vi "Main.vi"(9 "Device":string, 10 "VISA Com Port":refnum<visa-resource-name>, 11 "Module Admin":refnum<class "Delacor_lib_QMH_Cloneable Module Admin.lvclass">) -> ()   [LabVIEW 2020, in "Serial Device.lvlib"]
doc: "This template is based off of the Queued Message Handler design pattern and the Queued Message Handler project template that ships with LabVIEW.\n\nThe main difference is that the queue is private to this module and communication between modules is performed via Broadcast and Request events.\n\nRequest events are wrapped in public API methods and are handled in the Event Handling Loop (EHL) of this VI. Any module can register for Broadcast events sent by this module. The EHL generates messages based on user interface actions.\n\nThe Message Handling Loop (MHL) processes messages generated by the EHL, or by other messages. The messages are string values, so new messages can be added easily to the Message Cases case structure in the MHL. Each message cluster can also provide an optional value for Message Data, which is a variant that can be converted to whatever message-specific data is required.\n_____\nBased on Delacor QMH Project Template 5.0.0.82."
uses:
  Serial Device.lvlib
  <vilib>/Delacor/Delacor QMH/Libraries/Cloneable Module Admin_class/Delacor_lib_QMH_Cloneable Module Admin.lvclass
  C:/Program Files (x86)/National Instruments/LabVIEW 2020/vi.lib/Delacor/Delacor QMH/Libraries/Module Admin_class/Delacor_lib_QMH_Module Admin.lvclass
  Module Data--cluster.ctl
  <vilib>/Delacor/Delacor QMH/Libraries/Cloneable Module Admin_class/Delacor_lib_QMH_Cloneable Module Admin.lvclass/Delacor_lib_QMH_Cloneable Module Admin.ctl
  Stop Argument--cluster.ctl
  <vilib>/Delacor/Delacor QMH/Libraries/Message Queue_class/Delacor_lib_QMH_Message Queue.lvclass/Delacor_lib_QMH_Message Queue.ctl
  <vilib>/Delacor/Delacor QMH/Libraries/Module Admin_class/Delacor_lib_QMH_Module Admin.lvclass/Delacor_lib_QMH_Module Admin.ctl
  Write Port Argument--cluster.ctl
  Write Port (Reply Payload)--cluster.ctl
  Write Pin Argument--cluster.ctl
  Write Pin (Reply Payload)--cluster.ctl
  Read ADC Argument--cluster.ctl
  Read ADC (Reply Payload)--cluster.ctl
  Read Port Argument--cluster.ctl
  Read Port (Reply Payload)--cluster.ctl
  Read Pin Argument--cluster.ctl
  Read Pin (Reply Payload)--cluster.ctl
  Implementations/Cypress/Cypress.lvclass
  C:/Users/Asus/Dropbox/trabajos_apuntes/7 semestre/labview/Serial Device/Abstract/Serial Device/Serial Device.lvclass
  Implementations/Arduino/Arduino.lvclass
  Implementations/TI/TI.lvclass
  Implementations/Simulado/Simulado.lvclass
  Implementations/NXP/NXP.lvclass
  <vilib>/Utility/miscctls.llb/LVPointTypeDef.ctl
  <vilib>/Delacor/Delacor QMH/Libraries/Cloneable Module Admin_class/Delacor_lib_QMH_Get Module ID.vi
  <vilib>/Delacor/Delacor QMH/Libraries/Message Queue_class/Delacor_lib_QMH_Enqueue Message (Single).vi
  <vilib>/Delacor/Delacor QMH/Libraries/Module Admin_class/Delacor_lib_QMH_Get External Launch.vi
  <vilib>/Utility/error.llb/Error Cluster From Error Code.vi
  <vilib>/ErrorRing/Error Ring.xnode
  <vilib>/Delacor/Delacor QMH/Libraries/Message Queue_class/Delacor_lib_QMH_Message Queue.lvclass
  Abstract/Serial Device/Serial Device.lvclass
panel:
  out "Device Response":string
  in  "Read ADC":bool
  in  "Channel":dbl
  in  "Set Port":bool
  in  "Value":string="00"
  in  "Port":dbl
  out "Array":bool[](array[boolean])
  in  "Read Port":bool
  in  "Port 2":dbl caption="Port"
  in  "I/O Value":bool
  in  "Pin":dbl
  in  "Set PIN":bool
  in  "Port 3":dbl caption="Port"
  out "error out":errorcluster
  out "Pin Value":bool
  in  "Read PIN":bool
  in  "Pin 2":dbl caption="Pin"
  in  "Port 4":dbl caption="Port"
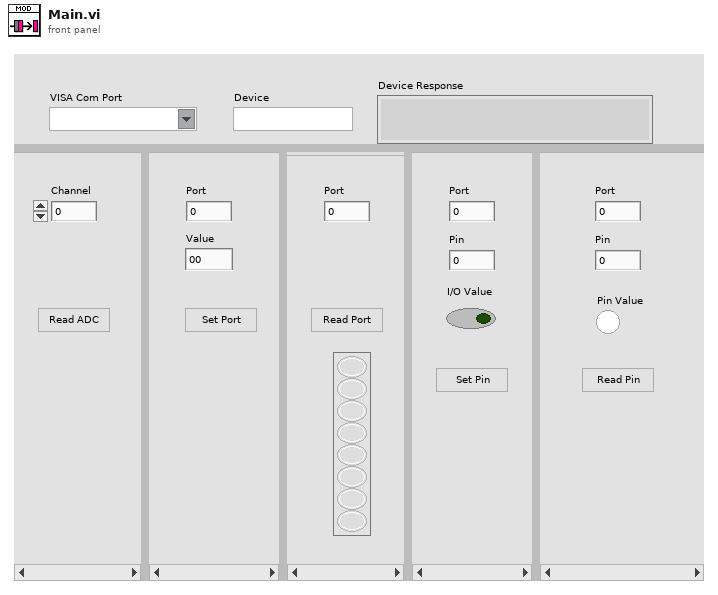
[diagram p1: front panel]
types:
  T1 = typedef "Serial Device.lvlib/Request Events--cluster.ctl" = cluster{"Stop Module":refnum<user-event>, "Show Panel":refnum<user-event>, "Hide Panel":refnum<user-event>, "Show Diagram":refnum<user-event>, "Get Module Execution Status":refnum<user-event>, "Write Port":refnum<user-event>, "Write Pin":refnum<user-event>, "Read ADC":refnum<user-event>, "Read Port":refnum<user-event>, "Read Pin":refnum<user-event>}
  T2 = typedef "Serial Device.lvlib/Module Data--cluster.ctl" = cluster{"Status":string}
  T3 = enum32{"invalid lock state", "Not Locked", "Locked (No Password)", "Password-protected"}
  T4 = typedef "Serial Device.lvlib/Stop Argument--cluster.ctl" = cluster{"Module ID":i32, "Origin":string, "Exit via Stop Module Req?":bool, "Wait for Module to stop?":bool}
  T5 = typedef "Serial Device.lvlib/Write Port Argument--cluster.ctl" = cluster{"Module ID":i32, "PORT":dbl, "VAL":string, "Wait Notifier":refnum<notifier>, "wait for reply":bool}
  T6 = typedef "Serial Device.lvlib/Write Pin Argument--cluster.ctl" = cluster{"Module ID":i32, "Port":dbl, "Value":bool, "Pin":dbl, "Wait Notifier":refnum<notifier>, "wait for reply":bool}
  T7 = typedef "Serial Device.lvlib/Read ADC Argument--cluster.ctl" = cluster{"Module ID":i32, "Channel":dbl, "Wait Notifier":refnum<notifier>, "wait for reply":bool}
  T8 = typedef "Serial Device.lvlib/Read Port Argument--cluster.ctl" = cluster{"Module ID":i32, "Port to read":dbl, "Wait Notifier":refnum<notifier>, "wait for reply":bool}
  T9 = typedef "Serial Device.lvlib/Read Pin Argument--cluster.ctl" = cluster{"Module ID":i32, "Port 4":dbl, "Pin 2":dbl, "Pin Value":bool, "Wait Notifier":refnum<notifier>, "wait for reply":bool}
  T10 = enum32{"Invalid", "Standard", "Closed", "Hidden", "Minimized", "Maximized"}
  T11 = typedef "Serial Device.lvlib/Write Port (Reply Payload)--cluster.ctl" = cluster{"Write Port_error":errorcluster, "Response":string}
  T12 = typedef "Serial Device.lvlib/Write Pin (Reply Payload)--cluster.ctl" = cluster{"Write Pin_error":errorcluster, "Response":string}
  T13 = typedef "Serial Device.lvlib/Read ADC (Reply Payload)--cluster.ctl" = cluster{"Read ADC_error":errorcluster, "Response":string}
  T14 = typedef "Serial Device.lvlib/Read Port (Reply Payload)--cluster.ctl" = cluster{"Read Port_error":errorcluster, "Response":string}
  T15 = typedef "Serial Device.lvlib/Read Pin (Reply Payload)--cluster.ctl" = cluster{"Read Pin_error":errorcluster, "Response":string}
  T16 = typedef "LVPointTypeDef.ctl" = cluster{"Horizontal":i16, "Vertical":i16}
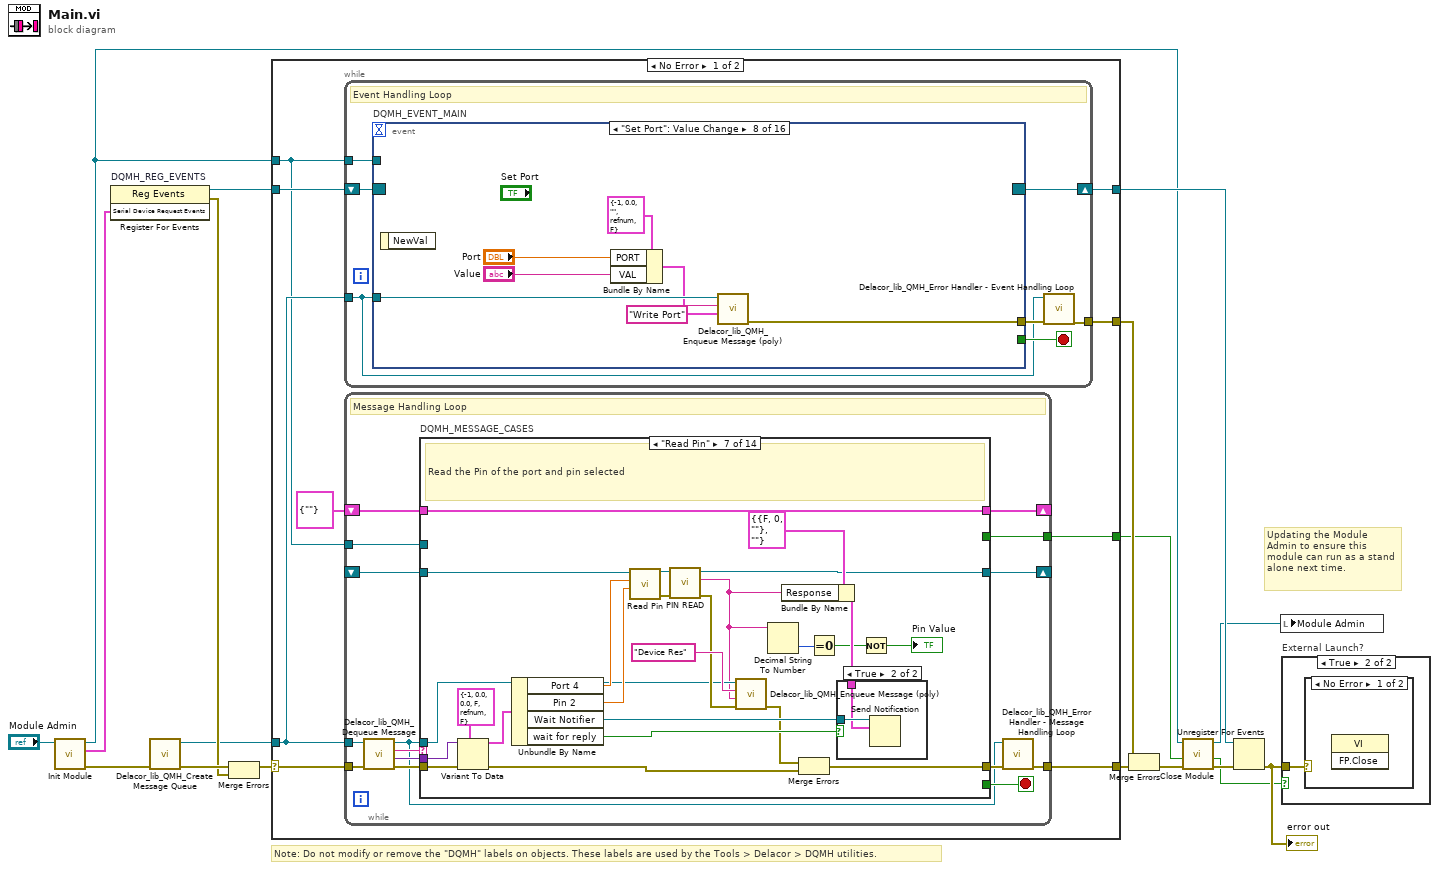
[diagram p0: block diagram]
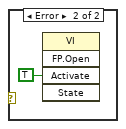
[diagram p3: hidden frame]
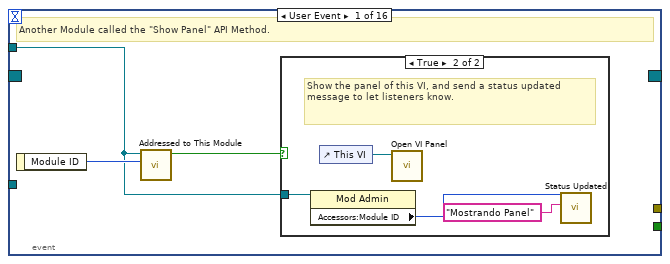
[diagram p4: hidden frame]
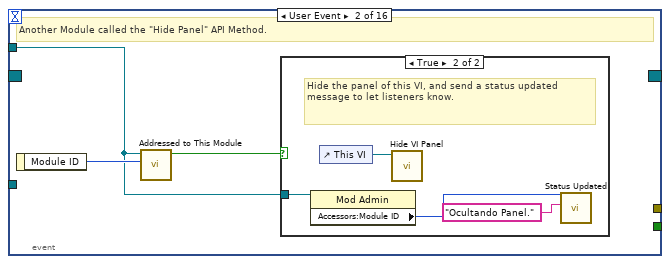
[diagram p6: hidden frame]
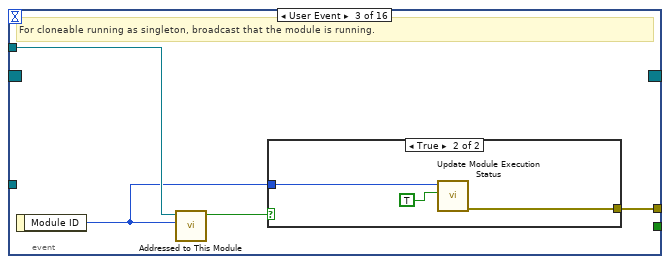
[diagram p8: hidden frame]
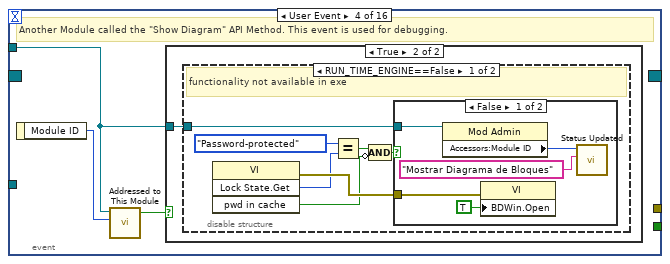
[diagram p10: hidden frame]
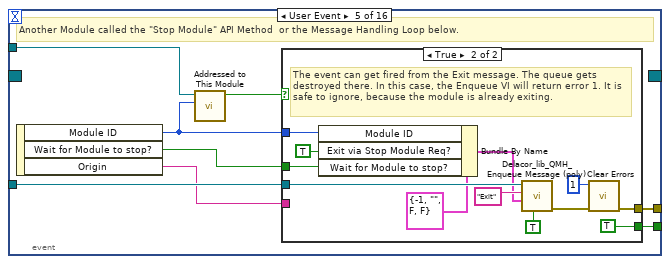
[diagram p14: hidden frame]
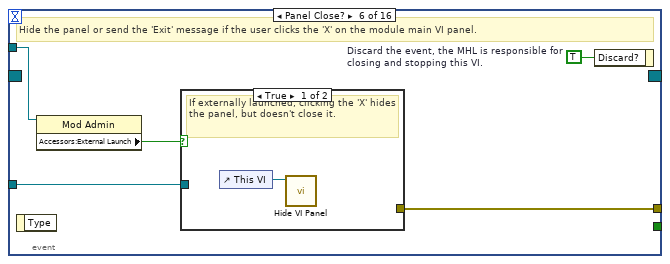
[diagram p16: hidden frame]
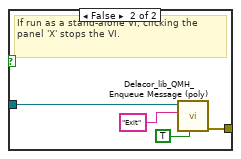
[diagram p17: hidden frame]
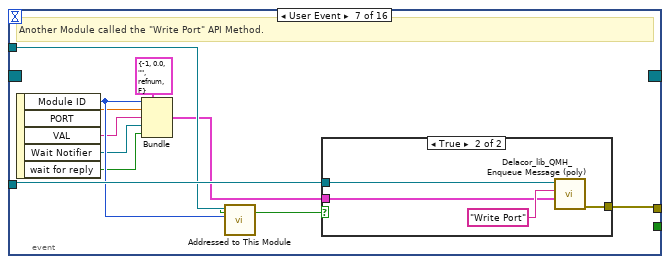
[diagram p18: hidden frame]
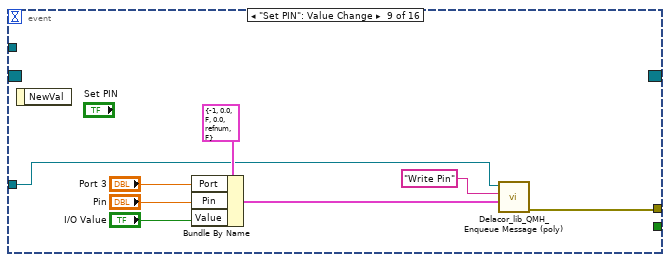
[diagram p20: hidden frame]
diagram:
  # "Note: Do not modify or remove the \"DQMH\" labels on objects. These labels are used by the Tools > Delacor > DQMH utilities."
  # "Updating the Module Admin to ensure this module can run as a stand alone next time."
  n1 = call "Init Module.vi"("Cloneable Module Admin in"="Module Admin") -> ("error out"=w15:errorcluster, "Serial Device Request Events"=w7:T1, "Cloneable Module Admin out"=w4:refnum<class "Delacor_lib_QMH_Cloneable Module Admin.lvclass">)  [unwired: 8 in]
  n2 = register-events "DQMH_REG_EVENTS"(w7) -> (reference out=w8:refnum<event-registration>, error out=w10:errorcluster)  [unwired: 2 in]
  n3 = call <vilib>:"Delacor_lib_QMH_Create Message Queue.vi"("error in (no error)"=w15) -> ("error out"=w12:errorcluster, "Message Queue"=w6:refnum<class "Delacor_lib_QMH_Message Queue.lvclass">)  [unwired: 9 in]
  n4 = Merge Errors(w12, w10) -> (w11:errorcluster)
  n5 = case shown="No Error" w11 {
    selector: w11 -> [w25 w478]
    tunnel: [w27 w477] -> w16
    tunnel: [w24 w485] -> w9
    tunnel: w8 -> [w22 w485]
    tunnel: w6 -> [w21 w476]
    tunnel: [w26 _] -> w17
    tunnel: w4 -> [w20 w481]
    tunnel: [w19 _] -> w2
    frame No Error {
      n6 = while {
        tunnel: w21 -> [w28]
        shift-right: [w31] -> w24
        shift-left: w22 -> [w32]
        tunnel: [w33] -> w26
        tunnel: w20 -> [w29]
        stop <- w30 stop-if-true
        # "Event Handling Loop"
        n7 = event "DQMH_EVENT_MAIN" shown="[7] \"Set Port\": Value Change" {
          selector: w32 -> [_ _ _ _ _ _ _ _ _ _ _ _ _ _ _ _]
          dyn-events: [_ _ _ _ _ _ _ _ _ _ _ _ _ _ _ _] -> w31
          timeout: _ -> [_ _ _ _ _ _ _ _ _ _ _ _ _ _ _ _]
          tunnel: [_ _ _ _ w75 _ _ _ _ _ _ _ _ _ _ _] -> w30
          tunnel: w28 -> [_ _ _ _ w78 w93 w112 w123 w126 w143 w157 w164 w177 w183 w190 w206]
          tunnel: [_ _ w52 _ w79 w96 w105 w122 w124 w134 w150 w163 w170 w184 w189 w197] -> w34
          tunnel: w29 -> [w35 w42 w50 w56 w77 w94 w111 _ _ w141 w155 _ w175 _ _ w204]
          event User Event {
            # "Another Module called the \"Show Panel\" API Method."
            n8 = event-data() -> ("Module ID"=w36:i32)  [unwired: 1 in]
            n9 = call "Addressed to This Module.vi"("Module ID from Argument"=w36, "Module Admin"=w35) -> ("Addressed to this instance?"=w37:bool)  [unwired: 8 in, 1 out]
            n10 = case shown="True" w37 {
              tunnel: w35 -> [_ w39]
              frame False {
              }
              frame True {
                # "Show the panel of this VI, and send a status updated message to let listeners know."
                n11 = property class="Mod Admin"(reference=w39) -> ("Accessors:Module ID"=w38:i32)  [unwired: 1 in, 2 out]
                n12 = control-ref of="This VI"() -> (w41:refnum<vi>)
                n13 = call "Open VI Panel.vi"("VI"=w41) -> ()  [unwired: 10 in, 1 out]
                n14 = call "Status Updated.vi"("Status"="Mostrando Panel" ("format string"), "Module ID"=w38) -> ()  [unwired: 9 in, 1 out]
              }
            }
          }
          event User Event {
            # "Another Module called the \"Hide Panel\" API Method."
            n15 = event-data() -> ("Module ID"=w43:i32)  [unwired: 1 in]
            n16 = call "Addressed to This Module.vi"("Module ID from Argument"=w43, "Module Admin"=w42) -> ("Addressed to this instance?"=w44:bool)  [unwired: 8 in, 1 out]
            n17 = case shown="True" w44 {
              tunnel: w42 -> [_ w46]
              frame False {
              }
              frame True {
                # "Hide the panel of this VI, and send a status updated message to let listeners know."
                n18 = property class="Mod Admin"(reference=w46) -> ("Accessors:Module ID"=w45:i32)  [unwired: 1 in, 2 out]
                n19 = control-ref of="This VI"() -> (w48:refnum<vi>)
                n20 = call "Hide VI Panel.vi"("VI"=w48) -> ()  [unwired: 10 in, 1 out]
                n21 = call "Status Updated.vi"("Status"="Ocultando Panel." ("format string"), "Module ID"=w45) -> ()  [unwired: 9 in, 1 out]
              }
            }
          }
          event User Event {
            # "For cloneable running as singleton, broadcast that the module is running."
            n22 = event-data() -> ("Module ID"=w49:i32)  [unwired: 1 in]
            n23 = call "Addressed to This Module.vi"("Module ID from Argument"=w49, "Module Admin"=w50) -> ("Addressed to this instance?"=w51:bool)  [unwired: 8 in, 1 out]
            n24 = case shown="True" w51 {
              tunnel: [_ w55] -> w52
              tunnel: w49 -> [_ w54]
              frame False {
              }
              frame True {
                n25 = call "Update Module Execution Status.vi"("Running?"=TRUE, "Module ID"=w54) -> ("error out"=w55:errorcluster)  [unwired: 9 in]
              }
            }
          }
          event User Event {
            # "Another Module called the \"Show Diagram\" API Method. This event is used for debugging."
            n26 = event-data() -> ("Module ID"=w57:i32)  [unwired: 1 in]
            n27 = call "Addressed to This Module.vi"("Module ID from Argument"=w57, "Module Admin"=w56) -> ("Addressed to this instance?"=w58:bool)  [unwired: 8 in, 1 out]
            n28 = case shown="True" w58 {
              tunnel: w56 -> [_ w59]
              frame False {
              }
              frame True {
                n29 = disable-structure shown="RUN_TIME_ENGINE==False" {
                  disable-tunnel: w59 -> [w60 _]
                  frame condition #0 (active) {
                    # "functionality not available in exe"
                    n30 = invoke class="VI" method="Lock State.Get"() -> (error out=w66:errorcluster, "Get Lock State"=w65:T3, "pwd in cache"=w62:bool)  [unwired: 4 in, 1 out]
                    n31 = Equal?(x=T3."Password-protected", y=w65) -> (x = y?=w63:bool)
                    n32 = Compound Arithmetic op=AND(w63, invert w62) -> (w61:bool)
                    n33 = case shown="False" w61 {
                      tunnel: w66 -> [w71 _]
                      tunnel: w60 -> [w68 _]
                      frame False {
                        n34 = property class="Mod Admin"(reference=w68) -> ("Accessors:Module ID"=w67:i32)  [unwired: 1 in, 2 out]
                        n35 = property class="VI"(error in=w71, "BDWin.Open"=TRUE ("Block Diagram Window:Open")) -> ()  [unwired: 1 in, 2 out]
                        n36 = call "Status Updated.vi"("Status"="Mostrar Diagrama de Bloques" ("format string"), "Module ID"=w67) -> ()  [unwired: 9 in, 1 out]
                      }
                      frame True {
                        # "Password-protected VI, and the password is not in the cache. Do not show the diagram."
                      }
                    }
                  }
                  frame condition #1 {
                  }
                }
              }
            }
          }
          event User Event {
            # "Another Module called the \"Stop Module\" API Method  or the Message Handling Loop below."
            n37 = event-data() -> ("Module ID"=w73:i32, "Wait for Module to stop?"=w74:bool, "Origin"=w72:string)  [unwired: 1 in]
            n38 = call "Addressed to This Module.vi"("Module ID from Argument"=w73, "Module Admin"=w77) -> ("Addressed to this instance?"=w76:bool)  [unwired: 8 in, 1 out]
            n39 = case shown="True" w76 {
              tunnel: [_ w90] -> w79
              tunnel: w78 -> [_ w86]
              tunnel: [_ TRUE] -> w75
              tunnel: w74 -> [_ w81]
              tunnel: w73 -> [_ w83]
              tunnel: w72 -> [_ _]
              frame False {
              }
              frame True {
                # "The event can get fired from the Exit message. The queue gets destroyed there. In this case, the Enqueue VI will return error 1. It is safe to ignore, because the module is already exiting."
                n40 = Bundle By Name(cluster=T4 {"Module ID"=-1, "Origin"="", "Exit via Stop Module Req?"=FALSE, "Wait for Module to stop?"=FALSE} ("Stop Argument"), "Module ID"=w83, "Exit via Stop Module Req?"=TRUE, "Wait for Module to stop?"=w81) -> (w80:T4)
                n41 = call-poly <vilib>:"Delacor_lib_QMH_Enqueue Message (poly).vi"("Priority Message? (F)"=TRUE, "Message Data"=w80, "Message"="Exit", "Message Queue in"=w86) -> ("error out"=w91:errorcluster)  [unwired: 6 in, 1 out]
                n42 = call <vilib>:"Clear Errors.vi"("error in (no error)"=w91, "specific error code to clear (0: all)"=1) -> ("error out"=w90:errorcluster)  [unwired: 4 in, 1 out]
              }
            }
          }
          event Panel Close? {
            w95 = TRUE  # Discard the event, the MHL is responsible for closing and stopping this VI.
            # "Hide the panel or send the 'Exit' message if the user clicks the 'X' on the module main VI panel."
            n43 = event-data() -> ()  [unwired: 1 in, 1 out]
            n44 = property class="Mod Admin"(reference=w94) -> ("Accessors:External Launch"=w92:bool)  [unwired: 1 in, 2 out]
            n45 = case shown="True" w92 {
              tunnel: w93 -> [_ w100]
              tunnel: [_ w101] -> w96
              frame True {
                # "If externally launched, clicking the 'X' hides the panel, but doesn't close it."
                n46 = control-ref of="This VI"() -> (w97:refnum<vi>)
                n47 = call "Hide VI Panel.vi"("VI"=w97) -> ()  [unwired: 10 in, 1 out]
              }
              frame False {
                # "If run as a stand-alone VI, clicking the panel 'X' stops the VI."
                n48 = call-poly <vilib>:"Delacor_lib_QMH_Enqueue Message (poly).vi"("Priority Message? (F)"=TRUE, "Message"="Exit", "Message Queue in"=w100) -> ("error out"=w101:errorcluster)  [unwired: 7 in, 1 out]
              }
            }
            n49 = event-data("Discard?"=w95) -> ()  [unwired: 1 in, 1 out]
          }
          event User Event {
            # "Another Module called the \"Write Port\" API Method."
            n50 = event-data() -> ("Module ID"=w108:i32, "PORT"=w107:dbl, "VAL"=w106:string, "Wait Notifier"=w104:refnum<notifier>, "wait for reply"=w103:bool)  [unwired: 1 in]
            n51 = Bundle(cluster=T5 {"Module ID"=-1, "PORT"=0.0, "VAL"="", "Wait Notifier"=refnum, "wait for reply"=FALSE} ("Write Port Argument"), "Module ID"=w108, "PORT"=w107, "VAL"=w106, "Wait Notifier"=w104, "wait for reply"=w103) -> (w109:T5)
            n52 = call "Addressed to This Module.vi"("Module ID from Argument"=w108, "Module Admin"=w111) -> ("Addressed to this instance?"=w102:bool)  [unwired: 8 in, 1 out]
            n53 = case shown="True" w102 {
              tunnel: w112 -> [_ w116]
              tunnel: w109 -> [_ w114]
              tunnel: [_ w113] -> w105
              frame False {
              }
              frame True {
                n54 = call-poly <vilib>:"Delacor_lib_QMH_Enqueue Message (poly).vi"("Message Data"=w114, "Message"="Write Port", "Message Queue in"=w116) -> ("error out"=w113:errorcluster)  [unwired: 7 in, 1 out]
              }
            }
          }
          event "Set Port": Value Change {
            n55 = event-data() -> ()  [unwired: 1 in, 1 out]
            n56 = Bundle By Name(cluster=T5 {"Module ID"=-1, "PORT"=0.0, "VAL"="", "Wait Notifier"=refnum, "wait for reply"=FALSE} ("Write Port Argument"), "PORT"="Port", "VAL"="Value") -> (w120:T5)
            n57 = call-poly <vilib>:"Delacor_lib_QMH_Enqueue Message (poly).vi"("Message Data"=w120, "Message"="Write Port", "Message Queue in"=w123) -> ("error out"=w122:errorcluster)  [unwired: 7 in, 1 out]
          }
          event "Set PIN": Value Change {
            n58 = event-data() -> ()  [unwired: 1 in, 1 out]
            n59 = Bundle By Name(cluster=T6 {"Module ID"=-1, "Port"=0.0, "Value"=FALSE, "Pin"=0.0, "Wait Notifier"=refnum, "wait for reply"=FALSE} ("Write Pin Argument"), "Port"="Port 3", "Pin"="Pin", "Value"="I/O Value") -> (w125:T6)
            n60 = call-poly <vilib>:"Delacor_lib_QMH_Enqueue Message (poly).vi"("Message Data"=w125, "Message"="Write Pin", "Message Queue in"=w126) -> ("error out"=w124:errorcluster)  [unwired: 7 in, 1 out]
          }
          event User Event {
            # "Another Module called the \"Write Pin\" API Method."
            n61 = event-data() -> ("Module ID"=w138:i32, "Port"=w137:dbl, "Value"=w136:bool, "Pin"=w135:dbl, "Wait Notifier"=w133:refnum<notifier>, "wait for reply"=w132:bool)  [unwired: 1 in]
            n62 = Bundle(cluster=T6 {"Module ID"=-1, "Port"=0.0, "Value"=FALSE, "Pin"=0.0, "Wait Notifier"=refnum, "wait for reply"=FALSE} ("Write Pin Argument"), "Module ID"=w138, "Port"=w137, "Value"=w136, "Pin"=w135, "Wait Notifier"=w133, "wait for reply"=w132) -> (w139:T6)
            n63 = call "Addressed to This Module.vi"("Module ID from Argument"=w138, "Module Admin"=w141) -> ("Addressed to this instance?"=w142:bool)  [unwired: 8 in, 1 out]
            n64 = case shown="True" w142 {
              tunnel: w143 -> [_ w147]
              tunnel: w139 -> [_ w145]
              tunnel: [_ w144] -> w134
              frame False {
              }
              frame True {
                n65 = call-poly <vilib>:"Delacor_lib_QMH_Enqueue Message (poly).vi"("Message Data"=w145, "Message"="Write Pin", "Message Queue in"=w147) -> ("error out"=w144:errorcluster)  [unwired: 7 in, 1 out]
              }
            }
          }
          event User Event {
            # "Another Module called the \"Read ADC\" API Method."
            n66 = event-data() -> ("Module ID"=w152:i32, "Channel"=w151:dbl, "Wait Notifier"=w149:refnum<notifier>, "wait for reply"=w148:bool)  [unwired: 1 in]
            n67 = Bundle(cluster=T7 {"Module ID"=-1, "Channel"=0.0, "Wait Notifier"=refnum, "wait for reply"=FALSE} ("Read ADC Argument"), "Module ID"=w152, "Channel"=w151, "Wait Notifier"=w149, "wait for reply"=w148) -> (w153:T7)
            n68 = call "Addressed to This Module.vi"("Module ID from Argument"=w152, "Module Admin"=w155) -> ("Addressed to this instance?"=w156:bool)  [unwired: 8 in, 1 out]
            n69 = case shown="True" w156 {
              tunnel: w157 -> [_ w161]
              tunnel: w153 -> [_ w159]
              tunnel: [_ w158] -> w150
              frame False {
              }
              frame True {
                n70 = call-poly <vilib>:"Delacor_lib_QMH_Enqueue Message (poly).vi"("Message Data"=w159, "Message"="Read ADC", "Message Queue in"=w161) -> ("error out"=w158:errorcluster)  [unwired: 7 in, 1 out]
              }
            }
          }
          event "Read ADC": Value Change {
            n71 = event-data() -> ()  [unwired: 1 in, 1 out]
            n72 = Bundle By Name(cluster=T7 {"Module ID"=-1, "Channel"=0.0, "Wait Notifier"=refnum, "wait for reply"=FALSE} ("Read ADC Argument"), "Channel"="Channel") -> (w162:T7)
            n73 = call-poly <vilib>:"Delacor_lib_QMH_Enqueue Message (poly).vi"("Message Data"=w162, "Message"="Read ADC", "Message Queue in"=w164) -> ("error out"=w163:errorcluster)  [unwired: 7 in, 1 out]
          }
          event User Event {
            # "Another Module called the \"Read Port\" API Method."
            n74 = event-data() -> ("Module ID"=w172:i32, "Port to read"=w171:dbl, "Wait Notifier"=w169:refnum<notifier>, "wait for reply"=w168:bool)  [unwired: 1 in]
            n75 = Bundle(cluster=T8 {"Module ID"=-1, "Port to read"=0.0, "Wait Notifier"=refnum, "wait for reply"=FALSE} ("Read Port Argument"), "Module ID"=w172, "Port to read"=w171, "Wait Notifier"=w169, "wait for reply"=w168) -> (w173:T8)
            n76 = call "Addressed to This Module.vi"("Module ID from Argument"=w172, "Module Admin"=w175) -> ("Addressed to this instance?"=w176:bool)  [unwired: 8 in, 1 out]
            n77 = case shown="True" w176 {
              tunnel: w177 -> [_ w181]
              tunnel: w173 -> [_ w179]
              tunnel: [_ w178] -> w170
              frame False {
              }
              frame True {
                n78 = call-poly <vilib>:"Delacor_lib_QMH_Enqueue Message (poly).vi"("Message Data"=w179, "Message"="Read Port", "Message Queue in"=w181) -> ("error out"=w178:errorcluster)  [unwired: 7 in, 1 out]
              }
            }
          }
          event "Read Port": Value Change {
            n79 = event-data() -> ()  [unwired: 1 in, 1 out]
            n80 = Bundle By Name(cluster=T8 {"Module ID"=-1, "Port to read"=0.0, "Wait Notifier"=refnum, "wait for reply"=FALSE} ("Read Port Argument"), "Port to read"="Port 2") -> (w182:T8)
            n81 = call-poly <vilib>:"Delacor_lib_QMH_Enqueue Message (poly).vi"("Message Data"=w182, "Message"="Read Port", "Message Queue in"=w183) -> ("error out"=w184:errorcluster)  [unwired: 7 in, 1 out]
          }
          event "Read PIN": Value Change {
            n82 = event-data() -> ()  [unwired: 1 in, 1 out]
            n83 = Bundle By Name(cluster=T9 {"Module ID"=-1, "Port 4"=0.0, "Pin 2"=0.0, "Pin Value"=FALSE, "Wait Notifier"=refnum, "wait for reply"=FALSE} ("Read Pin Argument"), "Port 4"="Port 4", "Pin 2"="Pin 2") -> (w188:T9)
            n84 = call-poly <vilib>:"Delacor_lib_QMH_Enqueue Message (poly).vi"("Message Data"=w188, "Message"="Read Pin", "Message Queue in"=w190) -> ("error out"=w189:errorcluster)  [unwired: 7 in, 1 out]
          }
          event User Event {
            # "Another Module called the \"Read Pin\" API Method."
            n85 = event-data() -> ("Module ID"=w201:i32, "Port 4"=w200:dbl, "Pin 2"=w199:dbl, "Pin Value"=w198:bool, "Wait Notifier"=w196:refnum<notifier>, "wait for reply"=w195:bool)  [unwired: 1 in]
            n86 = Bundle(cluster=T9 {"Module ID"=-1, "Port 4"=0.0, "Pin 2"=0.0, "Pin Value"=FALSE, "Wait Notifier"=refnum, "wait for reply"=FALSE} ("Read Pin Argument"), "Module ID"=w201, "Port 4"=w200, "Pin 2"=w199, "Pin Value"=w198, "Wait Notifier"=w196, "wait for reply"=w195) -> (w202:T9)
            n87 = call "Addressed to This Module.vi"("Module ID from Argument"=w201, "Module Admin"=w204) -> ("Addressed to this instance?"=w205:bool)  [unwired: 8 in, 1 out]
            n88 = case shown="True" w205 {
              tunnel: w206 -> [_ w210]
              tunnel: w202 -> [_ w208]
              tunnel: [_ w207] -> w197
              frame False {
              }
              frame True {
                n89 = call-poly <vilib>:"Delacor_lib_QMH_Enqueue Message (poly).vi"("Message Data"=w208, "Message"="Read Pin", "Message Queue in"=w210) -> ("error out"=w207:errorcluster)  [unwired: 7 in, 1 out]
              }
            }
          }
        }
        n90 = call-dynamic "Delacor_lib_QMH_Error Handler - Event Handling Loop.vi"("error in (no error)"=w34, "Message Queue in"=w28) -> ("dup error in"=w33:errorcluster)  [unwired: 8 in, 1 out]
      }
      n91 = while {
        tunnel: w21 -> [w216]
        shift-right: [w220] -> _
        shift-left: T2 {"Status"=""} ("Data Cluster") -> [w221]
        tunnel: w25 -> [w224]
        tunnel: [w222] -> w27
        tunnel: w20 -> [w214]
        tunnel: [w213] -> w19
        shift-right: [w212] -> _
        shift-left: _ -> [w211]
        stop <- w219 stop-if-true
        # "Message Handling Loop"
        n92 = call-dynamic "Delacor_lib_QMH_Dequeue Message.vi"("error in (no error)"=w224, "Message Queue in"=w216) -> ("error out"=w223:errorcluster, "Message Data"=w217:variant, "Message"=w218:string, "Message Queue out"=w215:refnum<class "Delacor_lib_QMH_Message Queue.lvclass">)  [unwired: 6 in]
        n93 = case "DQMH_MESSAGE_CASES" shown="\"Read Pin\"" w218 {
          selector: w218 -> [_ _ _ _ _ _ _ _ _ _ _ _ _ w463]
          tunnel: w215 -> [_ _ w266 w291 w317 _ w365 _ _ _ w405 _ w453 _]
          tunnel: w223 -> [w247 w262 w284 w312 w335 w357 w384 w390 w397 w400 w413 w433 w458 w465]
          tunnel: [w245 w262 w268 w302 w325 w347 w374 w389 w394 w400 w409 w432 w456 w466] -> w225
          tunnel: w221 -> [w238 w261 w283 w311 w334 w356 w383 w388 w396 w399 w402 w430 w452 w464]
          tunnel: [w237 w261 w283 w311 w334 w356 w383 w388 w396 w399 w402 w430 w452 w464] -> w220
          tunnel: [_ _ _ _ _ _ _ _ _ _ _ _ w451 _] -> w219
          tunnel: w217 -> [_ _ w282 w309 w332 w354 w381 _ w393 _ w408 _ w449 _]
          tunnel: w214 -> [w232 _ _ _ _ _ _ _ _ _ w407 w428 w445 w461]
          tunnel: [_ _ _ _ _ _ _ _ _ _ _ _ w447 _] -> w213
          tunnel: [w229 w260 w276 w295 w320 w343 w369 w387 w395 w398 w404 w426 w442 w459] -> w212
          tunnel: w211 -> [_ w260 w279 w296 w319 w342 w368 w387 w395 w398 w404 w426 w443 w459]
          frame "Initialize" {
            (unwired) T16 {"Horizontal"=0, "Vertical"=0} ("Origin")
            # "Initialize - Any operation that needs to be done before the module can receive messages. Synchronize Caller Events.vi will inform Start Module.vi that the module has launched and is ready to receive messages. Module Did Init.vi will broadcast that the module initialized."
            n94 = call "Synchronize Caller Events.vi"("error in (no error)"=w247, "Module Admin"=w232) -> ("error out"=w246:errorcluster, "Module Admin out"=w231:refnum<class "Delacor_lib_QMH_Cloneable Module Admin.lvclass">)  [unwired: 8 in]
            n95 = case shown="\"Simulado\", Default" "Device" {
              tunnel: [refnum<class "Cypress.lvclass"> refnum ("Cypress.lvclass") refnum<class "Arduino.lvclass"> refnum ("Arduino.lvclass") refnum<class "TI.lvclass"> refnum ("TI.lvclass") refnum<class "Simulado.lvclass"> refnum ("Simulado.lvclass") refnum<class "NXP.lvclass"> refnum ("NXP.lvclass")] -> w230
              tunnel: ["CY" ("read buffer") "AR" ("read buffer") "TI" ("read buffer") "SD" ("read buffer") "NX" ("read buffer")] -> w227
              frame "Cypress" {
              }
              frame "Arduino" {
              }
              frame "TI" {
              }
              frame "Simulado", Default {
              }
              frame "NXP" {
              }
            }
            n96 = property class="Mod Admin"(reference=w231) -> ("Accessors:Module ID"=w234:i32, "Accessors:External Launch"=w233:bool)  [unwired: 1 in, 2 out]
            n97 = call "Module Name--constant.vi"("Module ID"=w234) -> ("Module Name"=w242:string)  [unwired: 10 in]
            n98 = call-dynamic "Initialize.vi"("Device"=w227, "VISA Com Port"="VISA Com Port", "object in"=w230) -> ("object out"=w229:refnum<class "Serial Device.lvclass">)  [unwired: 7 in, 1 out]
            n99 = property class="VI"("Front Panel.Title"=w242) -> (reference out=w244:refnum<vi>, error out=w249:errorcluster)  [unwired: 2 in]
            n100 = Select(t=T10."Hidden" ("State"), s=w233, f=T10."Standard" ("State")) -> (s? t:f=w239:T10)
            n101 = invoke class="VI" method="FP.Open"(reference=w244, error in=w249, "State"=w239) -> (reference out=w243:refnum<vi>, error out=w248:errorcluster)  [unwired: 2 in, 3 out]
            n102 = Bundle By Name(cluster=w238, "Status"="Device") -> (w237:T2)
            n103 = call "Module Name--constant.vi"("Module ID"=w234) -> ("Module Name"=w235:string)  [unwired: 10 in]
            n104 = invoke class="VI" method="FP.Center"(reference=w243, error in=w248) -> ()  [unwired: 1 in, 3 out]
            n105 = call "Module Did Init.vi"("error in (no error)"=w246, "Initialized?"=TRUE, "Origin"=w235, "Module ID"=w234) -> ("error out"=w245:errorcluster)  [unwired: 7 in]
          }
          frame "--- Module Specific ---" {
            # "Separator -- The following cases handle messages specific to this Module."
          }
          frame "Write Port" {
            # "The user can modify the value of the Port that is linked into a bar led, the value must be in hex."
            n106 = Variant To Data(error in=w284, type=T5 {"Module ID"=-1, "PORT"=0.0, "VAL"="", "Wait Notifier"=refnum, "wait for reply"=FALSE} ("Write Port Argument"), Variant=w282) -> (data=w280:T5, error out=w272:errorcluster)
            n107 = Unbundle By Name(w280) -> ("PORT"=w273:dbl, "VAL"=w274:string, "wait for reply"=w265:bool, "Wait Notifier"=w264:refnum<notifier>)
            n108 = call-dynamic "Set Port Status.vi"("error in (no error)"=w272, "Value"=w274, "Port"=w273, "object in"=w279) -> ("error out"=w278:errorcluster, "object out"=w277:refnum<class "Serial Device.lvclass">)  [unwired: 6 in]
            n109 = call-dynamic "Read Command.vi"("error in (no error)"=w278, "Serial Device in"=w277) -> ("error out"=w271:errorcluster, "read buffer"=w263:string, "Serial Device out"=w276:refnum<class "Serial Device.lvclass">)  [unwired: 7 in]
            n110 = Bundle By Name(cluster=T11 {"Write Port_error"={"status"=FALSE, "code"=0, "source"=""}, "Response"=""} ("Write Port (Reply Payload)"), "Response"=w263) -> (w267:T11)
            n111 = case shown="True" w265 {
              tunnel: w264 -> [_ w289]
              tunnel: w271 -> [w285 w288]
              tunnel: [w285 w287] -> w269
              tunnel: w267 -> [_ w286]
              frame False {
              }
              frame True {
                n112 = Send Notification(notification=w286, notifier=w289, error in (no error)=w288) -> (error out=w287:errorcluster)  [unwired: 1 out]
              }
            }
            n113 = call-poly <vilib>:"Delacor_lib_QMH_Enqueue Message (poly).vi"("error in (no error)"=w269, "Message Data"=w263, "Message"="Device Res", "Message Queue in"=w266) -> ("error out"=w268:errorcluster)  [unwired: 6 in, 1 out]
          }
          frame "Write Pin" {
            # "In this Event the user can modify the status of each pin of the port selected"
            n114 = Variant To Data(error in=w312, type=T6 {"Module ID"=-1, "Port"=0.0, "Value"=FALSE, "Pin"=0.0, "Wait Notifier"=refnum, "wait for reply"=FALSE} ("Write Pin Argument"), Variant=w309) -> (data=w307:T6, error out=w310:errorcluster)
            n115 = Unbundle By Name(w307) -> ("Port"=w294:dbl, "Pin"=w293:dbl, "Value"=w292:bool, "Wait Notifier"=w306:refnum<notifier>, "wait for reply"=w305:bool)
            n116 = call-dynamic "Write Pin.vi"("Serial Device in"=w296, "Port"=w294, "Pin"=w293, "Value"=w292) -> ("Serial Device out"=w300:refnum<class "Serial Device.lvclass">, "error out"=w301:errorcluster)  [unwired: 10 in]
            n117 = call-dynamic "Read Command.vi"("error in (no error)"=w301, "Serial Device in"=w300) -> ("error out"=w299:errorcluster, "read buffer"=w297:string, "Serial Device out"=w295:refnum<class "Serial Device.lvclass">)  [unwired: 7 in]
            n118 = call-poly <vilib>:"Delacor_lib_QMH_Enqueue Message (poly).vi"("error in (no error)"=w299, "Message Data"=w297, "Message"="Device Res", "Message Queue in"=w291) -> ("error out"=w290:errorcluster)  [unwired: 6 in, 1 out]
            n119 = Bundle By Name(cluster=T12 {"Write Pin_error"={"status"=FALSE, "code"=0, "source"=""}, "Response"=""} ("Write Pin (Reply Payload)"), "Response"=w297) -> (w304:T12)
            n120 = Merge Errors(w290, w310) -> (w302:errorcluster)
            n121 = case shown="True" w305 {
              tunnel: w306 -> [_ w314]
              tunnel: w304 -> [_ w313]
              frame False {
              }
              frame True {
                n122 = Send Notification(notification=w313, notifier=w314) -> ()  [unwired: 1 in, 2 out]
              }
            }
          }
          frame "Read ADC" {
            # "Send the channel of the ADC to read and wait for the response of the Microcontroller"
            n123 = Variant To Data(error in=w335, type=T7 {"Module ID"=-1, "Channel"=0.0, "Wait Notifier"=refnum, "wait for reply"=FALSE} ("Read ADC Argument"), Variant=w332) -> (data=w330:T7, error out=w333:errorcluster)
            n124 = Unbundle By Name(w330) -> ("Channel"=w315:dbl, "Wait Notifier"=w329:refnum<notifier>, "wait for reply"=w328:bool)
            n125 = call-dynamic "Read ADC.vi"("ADC Channel"=w315, "object in"=w319) -> ("error out"=w323:errorcluster, "object out"=w324:refnum<class "Serial Device.lvclass">)  [unwired: 8 in]
            n126 = call-dynamic "Read Command.vi"("error in (no error)"=w323, "Serial Device in"=w324) -> ("error out"=w321:errorcluster, "read buffer"=w318:string, "Serial Device out"=w320:refnum<class "Serial Device.lvclass">)  [unwired: 7 in]
            n127 = call-poly <vilib>:"Delacor_lib_QMH_Enqueue Message (poly).vi"("error in (no error)"=w321, "Message Data"=w318, "Message"="Device Res", "Message Queue in"=w317) -> ("error out"=w316:errorcluster)  [unwired: 6 in, 1 out]
            n128 = Bundle By Name(cluster=T13 {"Read ADC_error"={"status"=FALSE, "code"=0, "source"=""}, "Response"=""} ("Read ADC (Reply Payload)"), "Response"=w318) -> (w327:T13)
            n129 = Merge Errors(w316, w333) -> (w325:errorcluster)
            n130 = case shown="True" w328 {
              tunnel: w329 -> [_ w337]
              tunnel: w327 -> [_ w336]
              frame False {
              }
              frame True {
                n131 = Send Notification(notification=w336, notifier=w337) -> ()  [unwired: 1 in, 2 out]
              }
            }
          }
          frame "Read Port" {
            # "The user can read an specific port that is selected from the UI of each instance"
            n132 = Variant To Data(error in=w357, type=T8 {"Module ID"=-1, "Port to read"=0.0, "Wait Notifier"=refnum, "wait for reply"=FALSE} ("Read Port Argument"), Variant=w354) -> (data=w352:T8, error out=w355:errorcluster)
            n133 = Unbundle By Name(w352) -> ("Port to read"=w340:dbl, "Wait Notifier"=w351:refnum<notifier>, "wait for reply"=w350:bool)
            n134 = call-dynamic "Port to Read.vi"("Port to Read"=w340, "Serial Device in"=w342) -> ("error out"=w346:errorcluster, "Serial Device out"=w345:refnum<class "Serial Device.lvclass">)  [unwired: 8 in]
            n135 = call-dynamic "Read Number.vi"("error in (no error)"=w346, "Serial Device in"=w345) -> ("error out"=w339:errorcluster, "Number Read"=w341:string, "Serial Device out"=w343:refnum<class "Serial Device.lvclass">)  [unwired: 7 in]
            n136 = Hexadecimal String To Number(string=w341) -> (number=w344:u32)  [unwired: 2 in, 1 out]
            n137 = Merge Errors(w339, w355) -> (w347:errorcluster)
            n138 = Number To Boolean Array(number=w344) -> (Boolean array=→"Array":bool[])
            n139 = Bundle By Name(cluster=T14 {"Read Port_error"={"status"=FALSE, "code"=0, "source"=""}, "Response"=""} ("Read Port (Reply Payload)"), "Response"=w341) -> (w349:T14)
            n140 = case shown="True" w350 {
              tunnel: w351 -> [_ w359]
              tunnel: w349 -> [_ w358]
              frame False {
              }
              frame True {
                n141 = Send Notification(notification=w358, notifier=w359) -> ()  [unwired: 1 in, 2 out]
              }
            }
          }
          frame "Read Pin" {
            # "Read the Pin of the port and pin selected"
            n142 = Variant To Data(error in=w384, type=T9 {"Module ID"=-1, "Port 4"=0.0, "Pin 2"=0.0, "Pin Value"=FALSE, "Wait Notifier"=refnum, "wait for reply"=FALSE} ("Read Pin Argument"), Variant=w381) -> (data=w379:T9, error out=w382:errorcluster)
            n143 = Unbundle By Name(w379) -> ("Port 4"=w367:dbl, "Pin 2"=w366:dbl, "Wait Notifier"=w378:refnum<notifier>, "wait for reply"=w377:bool)
            n144 = call-dynamic "Read Pin.vi"("Pin 2"=w366, "Port 4"=w367, "Serial Device in"=w368) -> ("error out"=w373:errorcluster, "Serial Device out"=w372:refnum<class "Serial Device.lvclass">)  [unwired: 7 in]
            n145 = call-dynamic "PIN READ.vi"("error in (no error)"=w373, "Serial Device in"=w372) -> ("error out"=w370:errorcluster, "VALUE"=w361:string, "Serial Device out"=w369:refnum<class "Serial Device.lvclass">)  [unwired: 7 in]
            n146 = call-poly <vilib>:"Delacor_lib_QMH_Enqueue Message (poly).vi"("error in (no error)"=w370, "Message Data"=w361, "Message"="Device Res", "Message Queue in"=w365) -> ("error out"=w364:errorcluster)  [unwired: 6 in, 1 out]
            n147 = Decimal String To Number(string=w361) -> (number=w363:i32)  [unwired: 2 in, 1 out]
            n148 = Bundle By Name(cluster=T15 {"Read Pin_error"={"status"=FALSE, "code"=0, "source"=""}, "Response"=""} ("Read Pin (Reply Payload)"), "Response"=w361) -> (w376:T15)
            n149 = Merge Errors(w364, w382) -> (w374:errorcluster)
            n150 = Equal To 0?(x=w363) -> (x = 0?=w362:bool)
            n151 = case shown="True" w377 {
              tunnel: w378 -> [_ w386]
              tunnel: w376 -> [_ w385]
              frame False {
              }
              frame True {
                n152 = Send Notification(notification=w385, notifier=w386) -> ()  [unwired: 1 in, 2 out]
              }
            }
            n153 = Not(x=w362) -> (.not. x?=→"Pin Value":bool)
          }
          frame "---Copy This Frame---" {
            # "Duplicate this frame when creating new messages.  Change this comment in the duplicated frame to describe this message."
            n154 = Merge Errors(w390) -> (w389:errorcluster)
          }
          frame "Device Res" {
            n155 = Variant To Data(error in=w397, type="", Variant=w393) -> (data=→"Device Response":string, error out=w394:errorcluster)
          }
          frame "--- Exit and Error Handling---" {
            # "Separator - the following cases handle errors and exit messages."
          }
          frame "Error" {
            # "Error - Check the error message data and respond accordingly. This message is sent by the \"Error Handler\" VIs at the end of each loop in this application."
            n156 = property class="Mod Admin"(reference=w407) -> ("Accessors:External Launch"=w406:bool, "Accessors:Module ID"=w403:i32)  [unwired: 1 in, 2 out]
            n157 = Variant To Data(error in=w413, type=errorcluster {"status"=FALSE, "code"=0, "source"=""} ("error constant"), Variant=w408) -> (data=w414:errorcluster, error out=w411:errorcluster)
            n158 = Unbundle By Name(w402) -> ("Status"=w401:string)
            n159 = call "Module Name--constant.vi"("Module ID"=w403) -> ()  [unwired: 10 in, 1 out]
            n160 = call "Error Reported.vi"("Additional Information"=w401, "Error"=w414, "Module ID"=w403) -> ()  [unwired: 8 in, 1 out]
            n161 = case shown="True" w406 {
              tunnel: [_ w425] -> w410
              tunnel: w405 -> [w417 w424]
              tunnel: w414 -> [w416 _]
              tunnel: w401 -> [_ w419]
              frame False {
                n162 = call <vilib>:"Simple Error Handler.vi"("error in (no error)"=w416) -> ()  [unwired: 4 in, 5 out]
                n163 = call-poly <vilib>:"Delacor_lib_QMH_Enqueue Message (poly).vi"("Priority Message? (F)"=TRUE, "Message"="Exit", "Message Queue in"=w417) -> ()  [unwired: 7 in, 2 out]
              }
              frame True {
                n164 = Concatenate Strings("Se perdio la conexión del dispositivo serial " ("message"), w419) -> (w421:string)
                n165 = call-poly <vilib>:"Delacor_lib_QMH_Enqueue Message (poly).vi"("Priority Message? (F)"=TRUE, "Message"="Exit", "Message Queue in"=w424) -> ("error out"=w425:errorcluster)  [unwired: 7 in, 1 out]
                n166 = One Button Dialog(message=w421) -> ()  [unwired: 1 in, 1 out]
              }
            }
            n167 = Merge Errors(w411, w410) -> (w409:errorcluster)
            n168 = local write "error out"(w409) -> ()
          }
          frame "Simulate MHL Error" {
            # "#DQMH_HowTo The 'Simulate MHL Error' button  illustrates how the MHL handles errors. This event is instructional in nature and can be removed."
            # "Simulate an error occurring at the MHL"
            n169 = property class="Mod Admin"(reference=w428) -> ("Accessors:Module ID"=w429:i32)  [unwired: 1 in, 2 out]
            n170 = call "Module Name--constant.vi"("Module ID"=w429) -> ("Module Name"=w427:string)  [unwired: 10 in]
            n171 = xnode "Error Ring"("parameter 0"=w427) -> ("error out"=w431:errorcluster)
            n172 = Merge Errors(w433, w431) -> (w432:errorcluster)
          }
          frame "Exit" {
            w450 = 91  # 91: not all Exit messages will have an argument
            w451 = TRUE  # Stop the VI
            # "Release the message queue reference"
            # "Exit - Exit the application."
            n173 = Variant To Data(error in=w458, type=T4 {"Module ID"=-1, "Origin"="", "Exit via Stop Module Req?"=FALSE, "Wait for Module to stop?"=FALSE} ("Stop Argument"), Variant=w449) -> (data=w446:T4, error out=w454:errorcluster)
            n174 = call <vilib>:"Clear Errors.vi"("error in (no error)"=w454, "specific error code to clear (0: all)"=w450) -> ("error out"=w457:errorcluster)  [unwired: 4 in, 1 out]
            n175 = call-dynamic "Delacor_lib_QMH_Release Message Queue.vi"("error in (no error)"=w457, "Message Queue"=w453) -> ("error out"=w441:errorcluster)  [unwired: 9 in]
            n176 = call-dynamic "Close Connection.vi"("object in"=w443) -> ("object out"=w442:refnum<class "Serial Device.lvclass">)  [unwired: 9 in, 1 out]
            n177 = control-ref of="This VI"() -> (w444:refnum<vi>)
            n178 = call "Handle Exit.vi"("Stop Argument"=w446, "Module Admin in"=w445, "VI reference"=w444) -> ("error out"=w455:errorcluster, "Wait for Stop?"=w447:bool)  [unwired: 7 in]
            n179 = Merge Errors(w455, w441) -> (w456:errorcluster)
          }
          frame Default {
            # "'Default' case only runs if there is a message that isn't defined in any of the other cases.  Output a programming error."
            n180 = property class="Mod Admin"(reference=w461) -> ("Accessors:Module ID"=w460:i32)  [unwired: 1 in, 2 out]
            n181 = call "Module Name--constant.vi"("Module ID"=w460) -> ("Module Name"=w462:string)  [unwired: 10 in]
            n182 = xnode "Error Ring"("parameter 0"=w463, "parameter 1"=w462) -> ("error out"=w467:errorcluster)
            n183 = Merge Errors(w465, w467) -> (w466:errorcluster)
          }
        }
        n184 = call-dynamic "Delacor_lib_QMH_Error Handler - Message Handling Loop.vi"("error in (no error)"=w225, "Message Queue in"=w215) -> ("dup error in"=w222:errorcluster)  [unwired: 8 in, 1 out]
      }
    }
    frame Error {
      n185 = call "Synchronize Caller Events.vi"("Module Admin"=w481) -> ("Module Admin out"=w480:refnum<class "Delacor_lib_QMH_Cloneable Module Admin.lvclass">)  [unwired: 9 in, 1 out]
      n186 = property class="Mod Admin"(reference=w480) -> ("Accessors:Module ID"=w479:i32)  [unwired: 1 in, 2 out]
      n187 = call-dynamic "Delacor_lib_QMH_Release Message Queue.vi"("error in (no error)"=w478, "Message Queue"=w476) -> ("error out"=w477:errorcluster)  [unwired: 9 in]
      n188 = call "Module Name--constant.vi"("Module ID"=w479) -> ("Module Name"=w484:string)  [unwired: 10 in]
      n189 = Format Into String(format string="An error occurred during initialization. %s is no longer running.", w484) -> (resulting string=w482:string)  [unwired: 2 in, 1 out]
      n190 = call "Error Reported.vi"("Additional Information"=w482, "Error"=w477, "Module ID"=w479) -> ()  [unwired: 8 in, 1 out]
    }
  }
  n191 = Merge Errors(w17, w16) -> (w18:errorcluster)
  n192 = call "Close Module.vi"("error in"=w18, "Wait for stop?"=w2, "Module Admin in"=w4) -> ("error out"=w14:errorcluster, "External Launch"=w1:bool, "Module Admin out"=w3:refnum<class "Delacor_lib_QMH_Cloneable Module Admin.lvclass">)  [unwired: 6 in]
  n193 = Unregister For Events(event registration refnum=w9, error in=w14) -> (error out=w13:errorcluster)
  "error out" <- w13
  n194 = local write "Module Admin"(w3) -> ()
  n195 = case "External Launch?" shown="True" w1 {
    tunnel: w13 -> [_ w486]
    frame False {
    }
    frame True {
      n196 = case shown="No Error" w486 {
        frame No Error {
          n197 = invoke class="VI" method="FP.Close"() -> ()  [unwired: 3 in, 3 out]
        }
        frame Error {
          n198 = invoke class="VI" method="FP.Open"("Activate"=TRUE ("Activate?")) -> ()  [unwired: 4 in, 5 out]
        }
      }
    }
  }
